vi "test query_parts.vi"() -> ()   [LabVIEW 2017]
uses:
  DB Part.ctl
  Database.lvlib
panel:
  out "Parts":T1[](array[typedef])
  out "error out":errorcluster
  in  "port":i32=33060
  in  "host":string="localhost"
  in  "password":string="carriker"
  in  "username":string="root"
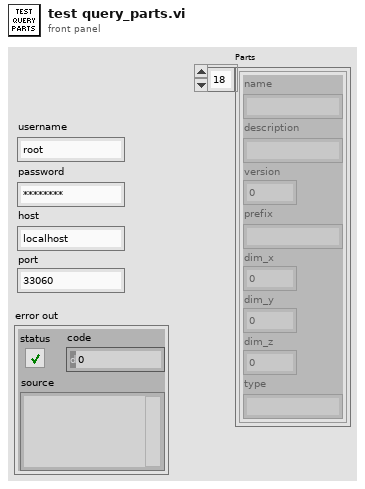
[diagram p1: front panel]
types:
  T1 = typedef "Database.lvlib/DB Part.ctl" = cluster{"name":string, "description":string, "version":i32, "prefix":string, "dim_x":sgl, "dim_y":sgl, "dim_z":sgl, "type":string}
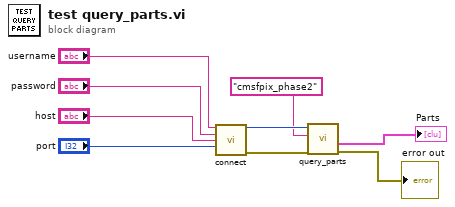
[diagram p0: block diagram]
diagram:
  n1 = call "connect.vi"("username"="username", "password"="password", "host"="host", "port"="port") -> ("DB Session ID"=w5:i32, "error out"=w4:errorcluster)  [unwired: 10 in]
  n2 = call "query_parts.vi"("error in (no error)"=w4, "Schema"="cmsfpix_phase2", "DB Session ID"=w5) -> ("error out"=→"error out":errorcluster, "Parts"=→"Parts":T1[])  [unwired: 5 in, 2 out]
